vi "Login.vi"() -> ()   [LabVIEW 2015]
uses:
  Queues and Variants 8.2/Queue Element.ctl
  Queues and Variants 8.2/Data Type.ctl
  <vilib>/httpClient/LabVIEWHTTPClient.lvlib
panel:
  in  "OK Button 4":bool
  in  "OK Button 3":bool
  in  "OK Button 2":bool
  out "Tab Control 2":enum32{"Page 1", "Page 2"}(tab)
  out "Tab Control":enum32{"Page 1", "Page 2"}(tab)
  in  "OK Button":bool
  in  "String 2":string
  in  "String":string
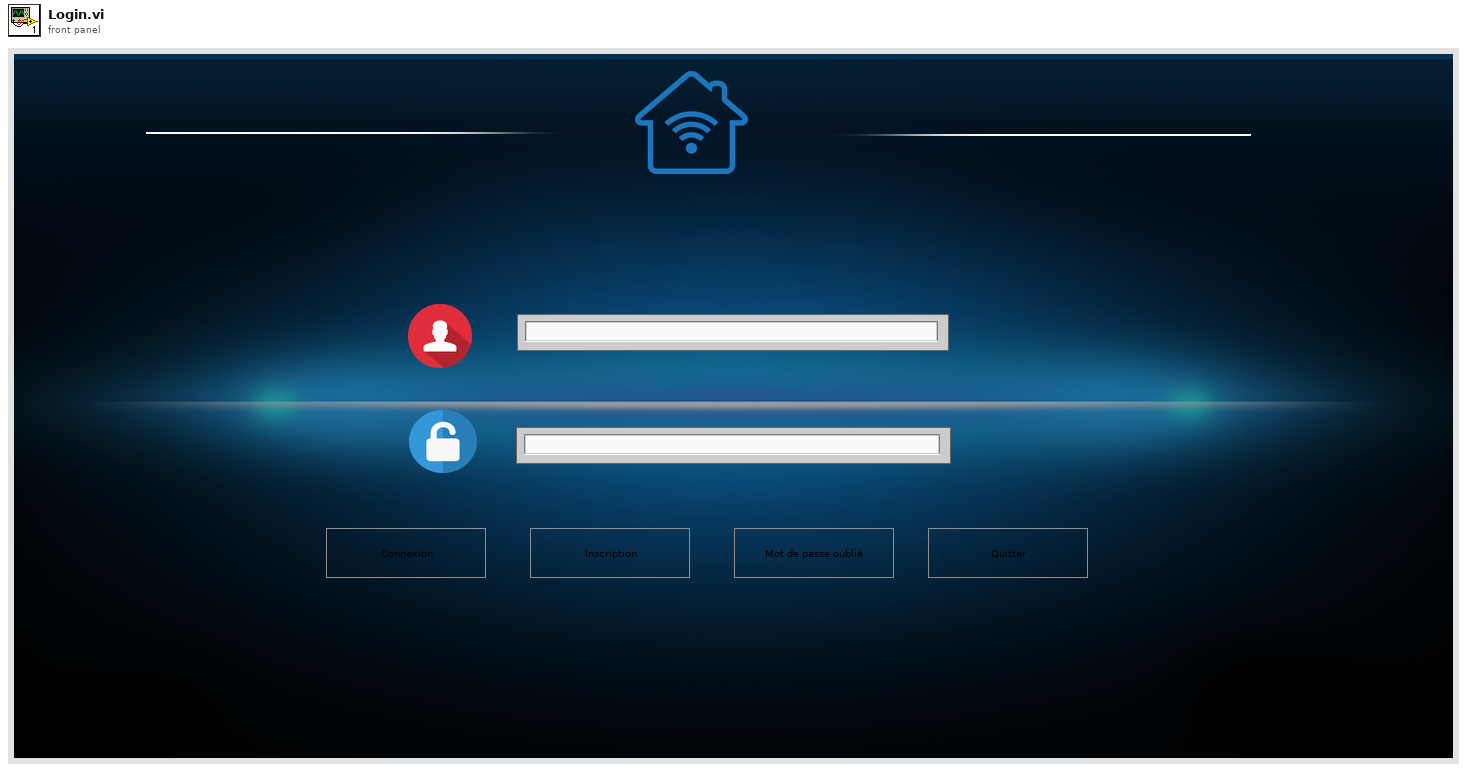
[diagram p1: front panel]
types:
  T1 = typedef "Data Type.ctl" = enum16{"Double Precision", "String", "Boolean"}
  T2 = typedef "Queue Element.ctl" = cluster{"Data Type":T1, "Variant":variant}
  T3 = enum32{"Invalid", "Standard", "Closed", "Hidden", "Minimized", "Maximized"}
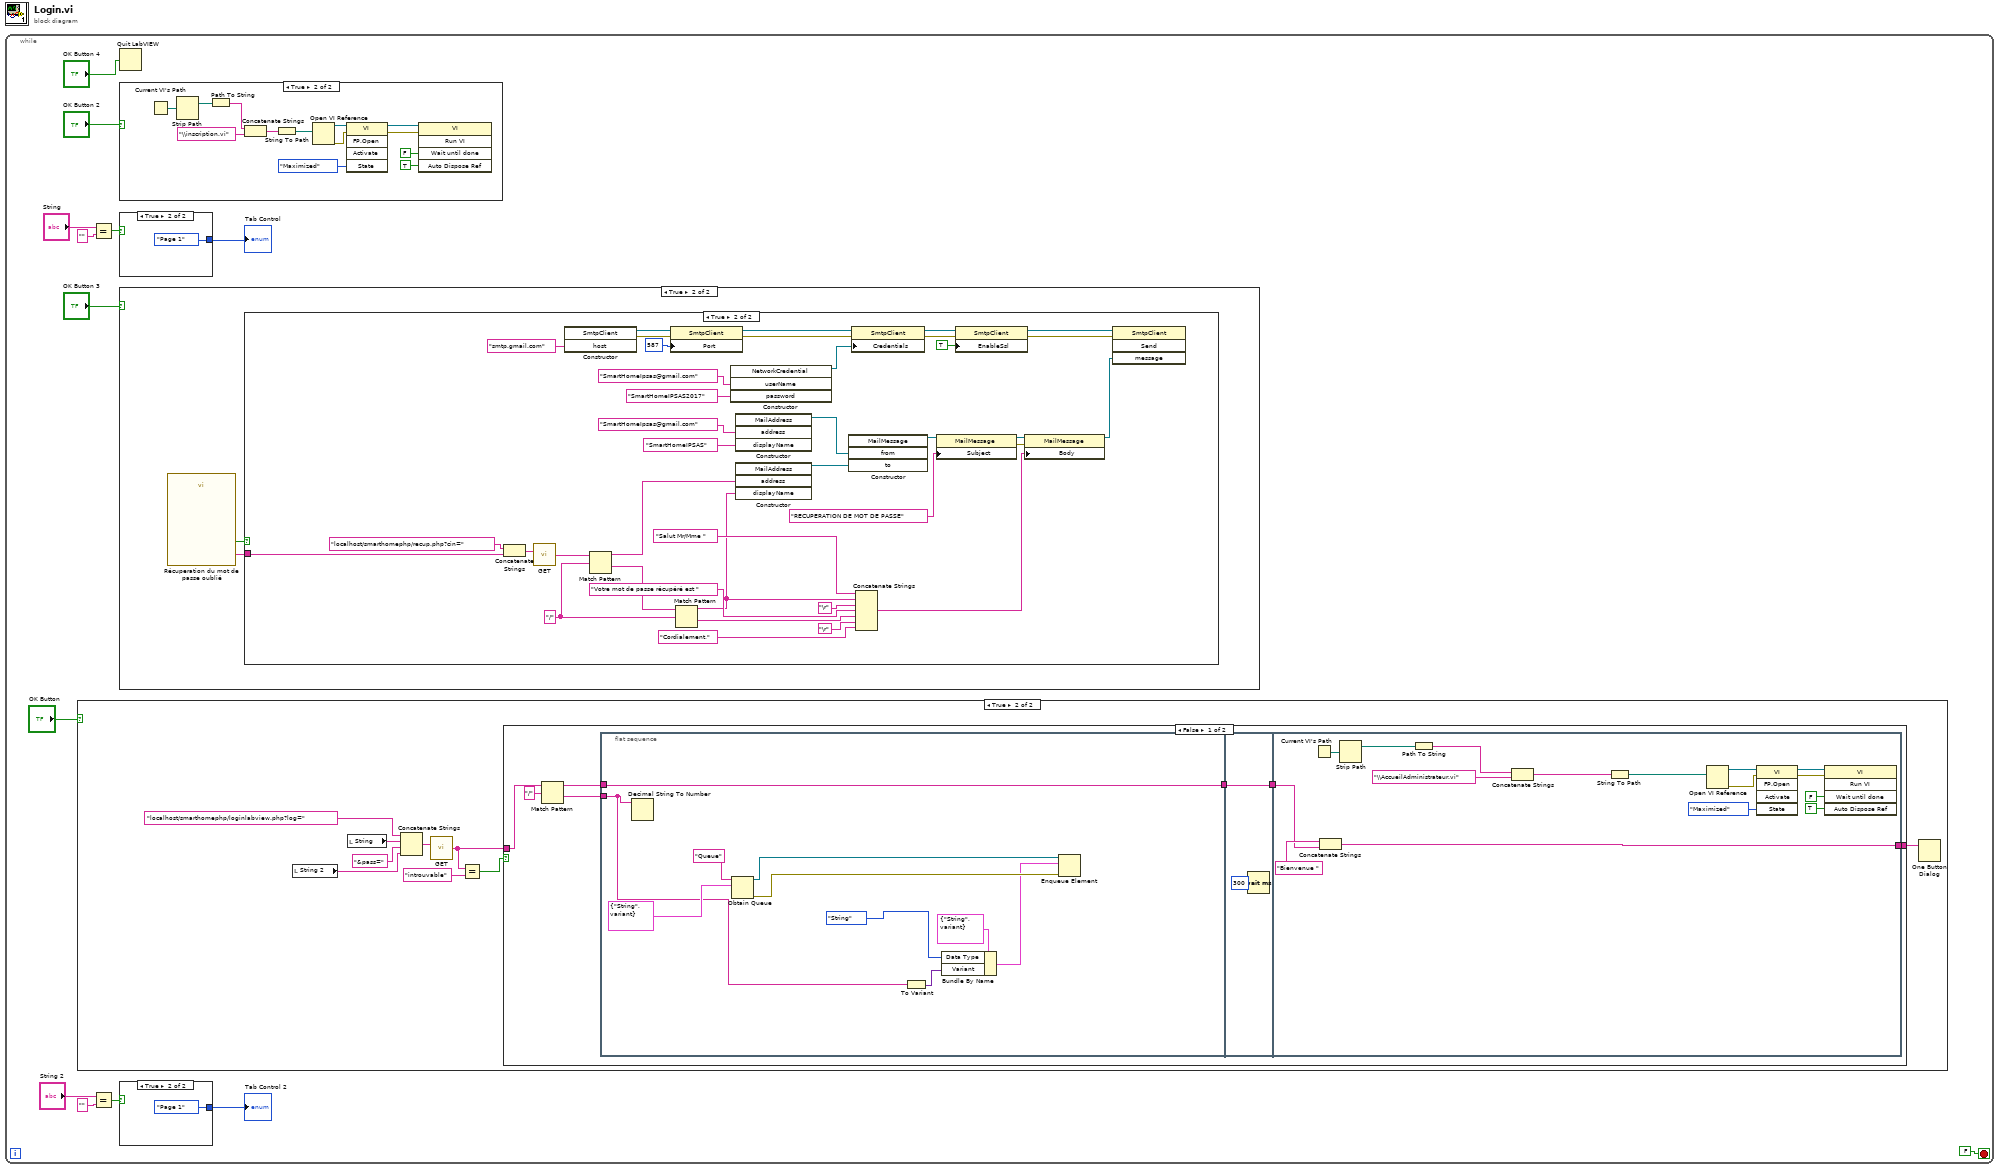
[diagram p0: block diagram]
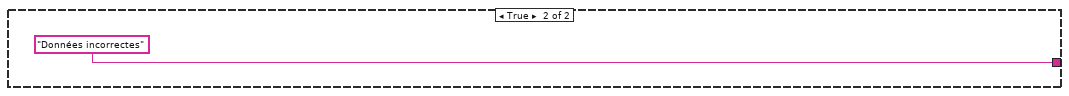
[diagram p5: hidden frame]
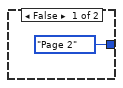
[diagram p7: hidden frame]
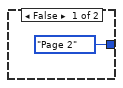
[diagram p8: hidden frame]
diagram:
  n1 = while {
    stop <- FALSE stop-if-true
    n2 = case shown="True" "OK Button" {
      frame False {
      }
      frame True {
        n3 = local read "String 2"() -> (w59:string)
        n4 = local read "String"() -> (w61:string)
        n5 = Concatenate Strings("localhost/smarthomephp/loginlabview.php?log=", w61, "&pass=", w59) -> (w58:string)
        n6 = call <vilib>:"GET.vi"("url"=w58) -> ("body"=w55:string)  [unwired: 11 in, 3 out]
        n7 = Equal?(x=w55, y="introuvable") -> (x = y?=w56:bool)
        n8 = case shown="False" w56 {
          tunnel: w55 -> [w67 _]
          tunnel: [w69 "Données incorrectes"] -> w54
          frame False {
            n9 = Match Pattern(string=w67, regular expression="/") -> (before substring=w68:string, after substring=w65:string)  [unwired: 1 in, 2 out]
            n10 = flat-sequence {
              tunnel: w68 -> [w79]
              tunnel: [w79] -> w64
              tunnel: w65 -> [w72]
              tunnel: w64 -> [w81]
              tunnel: [w81] -> w63
              tunnel: [w96] -> w69
              tunnel: w63 -> [w82]
              frame #0 {
                n11 = Decimal String To Number(string=w72) -> ()  [unwired: 2 in, 2 out]
                n12 = Obtain Queue(name (unnamed)="Queue", element data type=T2 {"Data Type"=enum."String", "Variant"=variant} ("Queue Element")) -> (queue out=w75:refnum<queue>, error out=w76:errorcluster)  [unwired: 3 in, 1 out]
                n13 = To Variant(anything=w72) -> (Variant=w70:variant)
                n14 = Bundle By Name(cluster=T2 {"Data Type"=enum."String", "Variant"=variant} ("Queue Element"), "Data Type"=Data_Type."String" ("Data Type 2"), "Variant"=w70) -> (w73:T2)
                n15 = Enqueue Element(queue=w75, element=w73, error in (no error)=w76) -> ()  [unwired: 4 out]
              }
              frame #1 {
                n16 = Wait (ms)(milliseconds to wait=u32 300) -> ()  [unwired: 1 out]
              }
              frame #2 {
                n17 = Current VI's Path() -> (path=w83:path)
                n18 = Concatenate Strings("Bienvenue ", w82) -> (w96:string)
                n19 = Strip Path(path=w83) -> (stripped path=w84:path)  [unwired: 1 out]
                n20 = Path To String(path=w84) -> (string=w85:string)
                n21 = Concatenate Strings(w85, "\\AccueilAdministrateur.vi") -> (w87:string)
                n22 = String To Path(string=w87) -> (path=w88:path)
                n23 = Open VI Reference(vi path=w88) -> (vi reference=w89:refnum<vi>, error out=w90:errorcluster)  [unwired: 5 in]
                n24 = invoke class="VI" method="FP.Open"(reference=w89, error in=w90, "State"=T3."Maximized") -> (reference out=w91:refnum<vi>, error out=w92:errorcluster)  [unwired: 2 in, 3 out]
                n25 = invoke class="VI" method="Run VI"(reference=w91, error in=w92, "Wait until done"=FALSE ("Wait Until Done"), "Auto Dispose Ref"=TRUE ("Auto Dispose Reference")) -> ()  [unwired: 1 in, 5 out]
              }
            }
          }
          frame True {
          }
        }
        n26 = One Button Dialog(message=w54) -> ()  [unwired: 1 in, 1 out]
      }
    }
    n27 = Equal?(x="String", y="") -> (x = y?=w9:bool)
    n28 = Equal?(x="String 2", y="") -> (x = y?=w8:bool)
    n29 = Quit LabVIEW(quit? (T)="OK Button 4") -> ()
    n30 = case shown="True" "OK Button 2" {
      frame False {
      }
      frame True {
        n31 = Current VI's Path() -> (path=w111:path)
        n32 = Strip Path(path=w111) -> (stripped path=w110:path)  [unwired: 1 out]
        n33 = Path To String(path=w110) -> (string=w109:string)
        n34 = Concatenate Strings(w109, "\\inscription.vi") -> (w107:string)
        n35 = String To Path(string=w107) -> (path=w106:path)
        n36 = Open VI Reference(vi path=w106) -> (vi reference=w105:refnum<vi>, error out=w104:errorcluster)  [unwired: 5 in]
        n37 = invoke class="VI" method="FP.Open"(reference=w105, error in=w104, "State"=T3."Maximized") -> (reference out=w103:refnum<vi>, error out=w102:errorcluster)  [unwired: 2 in, 3 out]
        n38 = invoke class="VI" method="Run VI"(reference=w103, error in=w102, "Wait until done"=FALSE ("Wait Until Done"), "Auto Dispose Ref"=TRUE ("Auto Dispose Reference")) -> ()  [unwired: 1 in, 5 out]
      }
    }
    n39 = case shown="True" w9 {
      tunnel: [enum32{"Page 1", "Page 2"}."Page 2" ("Tab Control") enum32{"Page 1", "Page 2"}."Page 1" ("Tab Control")] -> w6
      frame False {
      }
      frame True {
      }
    }
    "Tab Control" <- w6
    n40 = case shown="True" "OK Button 3" {
      frame False {
      }
      frame True {
        n41 = call "Récuperation du mot de passe oublié"() -> ("Entrer votre CIN:"=w14:string, "Récupération"=w15:bool)  [unwired: 17 in, 1 out]
        n42 = case shown="True" w15 {
          tunnel: w14 -> [_ w52]
          frame False {
          }
          frame True {
            w48 = "/" ("regular expression")
            n43 = Concatenate Strings("localhost/smarthomephp/recup.php?cin=", w52) -> (w51:string)
            n44 = call <vilib>:"GET.vi"("url"=w51) -> ("body"=w50:string)  [unwired: 11 in, 3 out]
            n45 = constructor class="SmtpClient"("host"="smtp.gmail.com" ("Outgoing Mail Server (SMTP)")) -> (reference out=w34:refnum<k24>, error out=w30:errorcluster)  [unwired: 3 in, 2 out]
            n46 = Match Pattern(string=w50, regular expression=w48) -> (before substring=w24:string, after substring=w49:string)  [unwired: 1 in, 2 out]
            n47 = property class="SmtpClient"(reference=w34, error in=w30, "Port"=587) -> (reference out=w33:refnum<k24>, error out=w29:errorcluster)
            n48 = Match Pattern(string=w49, regular expression=w48) -> (before substring=w20:string, after substring=w19:string)  [unwired: 1 in, 2 out]
            n49 = constructor class="NetworkCredential"("userName"="SmartHomeIpsas@gmail.com" ("GMAIL Account User ID (eg: jsmity77)"), "password"="SmartHomeIPSAS2017" ("GMAIL Account Password")) -> (reference out=w35:refnum<k24>)  [unwired: 3 in, 4 out]
            n50 = constructor class="MailAddress"("address"="SmartHomeIpsas@gmail.com" ("Sender's Email Address (eg: jsmith77@gmail.com)"), "displayName"="SmartHomeIPSAS" ("Sender's Name")) -> (reference out=w46:refnum<k24>)  [unwired: 3 in, 4 out]
            n51 = constructor class="MailAddress"("address"=w24, "displayName"=w20) -> (reference out=w47:refnum<k24>)  [unwired: 3 in, 4 out]
            n52 = constructor class="MailMessage"("from"=w46, "to"=w47) -> (reference out=w26:refnum<k24>)  [unwired: 3 in, 4 out]
            n53 = property class="SmtpClient"(reference=w33, error in=w29, "Credentials"=w35) -> (reference out=w32:refnum<k24>, error out=w28:errorcluster)
            n54 = Concatenate Strings("Salut Mr/Mme " ("Body"), w20, "\r", "Votre mot de passe récupéré est " ("Body"), w19, "\r", "Cordialement," ("string")) -> (w16:string)
            n55 = property class="MailMessage"(reference=w26, "Subject"="RECUPERATION DE MOT DE PASSE") -> (reference out=w40:refnum<k24>, error out=w45:errorcluster)  [unwired: 1 in]
            n56 = property class="SmtpClient"(reference=w32, error in=w28, "EnableSsl"=TRUE ("Enable SSL")) -> (reference out=w31:refnum<k24>, error out=w27:errorcluster)
            n57 = property class="MailMessage"(reference=w40, error in=w45, "Body"=w16) -> (reference out=w25:refnum<k24>)  [unwired: 1 out]
            n58 = invoke class="SmtpClient" method="Send"(reference=w31, error in=w27, "message"=w25) -> ()  [unwired: 1 in, 4 out]
          }
        }
      }
    }
    n59 = case shown="True" w8 {
      tunnel: [enum32{"Page 1", "Page 2"}."Page 2" ("Tab Control") enum32{"Page 1", "Page 2"}."Page 1" ("Tab Control")] -> w7
      frame False {
      }
      frame True {
      }
    }
    "Tab Control 2" <- w7
  }
